vi "Test Copy from Pixmap Offset.vi"(8 "error in (no error)":errorcluster, 11 "Test Case In":refnum<class "Image.lvclass">) -> (0 "error out":errorcluster, 3 "Test Case Out":refnum<class "Image.lvclass">)   [LabVIEW 2020, in "g_ar_toolkit.test.lvlib" / "Image.lvclass"]
uses:
  Image.lvclass
  C:/Program Files (x86)/National Instruments/LabVIEW 2020/vi.lib/Astemes/LUnit/Test Case.lvclass
  g_ar_toolkit.image/ARGB Colour.ctl
  <vilib>/Astemes/LUnit/Test Case.lvclass/Test Case.ctl
  g_ar_toolkit.image/CreateEmptyImageARGB.vi
  g_ar_toolkit.image/CopyPixmapToImageFlattenMaskARGB.vi
  4993e8ee-a06a-463a-9684-69129f64d5ce.vi
  g_ar_toolkit.image/CreateEmptyImageARGB.vi/3321fa97-f432-4e1e-8db9-a0df79aed21b.vi
  g_ar_toolkit.image/CopyPixmapToImageFlattenMaskARGB.vi/80b1166a-8c06-443b-b271-eb6a715622f7.vi
  <vilib>/Astemes/LUnit/Append Pass Result.vi
  <vilib>/Astemes/LUnit/Append Fail Result.vi
  <vilib>/Astemes/LUnit/Describe Comparison.vi
  <vilib>/Astemes/LUnit/Compare Variants.vi
  g_ar_toolkit.image/FixPixmap.vi
  <vilib>/Astemes/LUnit/Run In UI.vi
  g_ar_toolkit.image/Default8bitColourMap.vi
  <vilib>/Utility/error.llb/Clear Errors.vi
  g_ar_toolkit.image/ARGBColourToU32.vi
  g_ar_toolkit.common/Module Path.vi
  <vilib>/Utility/error.llb/Error Cluster From Error Code.vi
  <vilib>/Astemes/LUnit/Describe Variant.vi
  g_ar_toolkit.image/g_ar_toolkit.image.lvlib
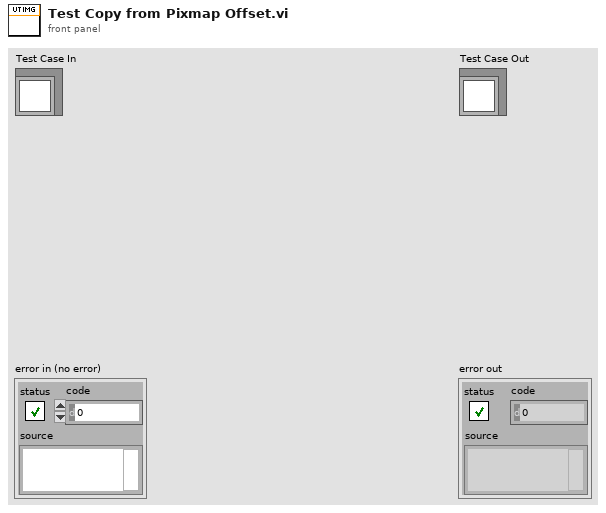
[diagram p1: front panel]
types:
  T1 = cluster{"Width":i16, "Style":enum32{"Solid", "Dash", "Dot", "DashDot", "DashDotDot"}}
  T2 = typedef "g_ar_toolkit.image.lvlib/ARGB Colour.ctl" = cluster{"Alpha":u8, "RGB":u32}
  T3 = cluster{"left":i16, "top":i16, "right":i16, "bottom":i16}
  T4 = typedef "imagedata.ctl" = cluster{"image type":i32, "image depth":i32, "image":u8[], "mask":u8[], "colors":u32[], "Rectangle":cluster{"left":i16, "top":i16, "right":i16, "bottom":i16}}
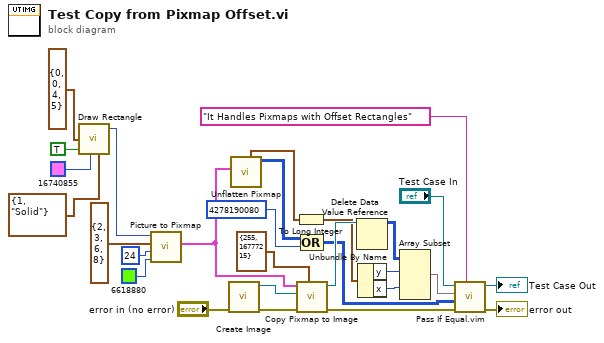
[diagram p0: block diagram]
diagram:
  n1 = call <vilib>:"Draw Rectangle.vi"("rect"=T3 {"left"=0, "top"=0, "right"=4, "bottom"=5}, "fill?(F)"=TRUE, "color(black)"=u32 16740855, "pen"=T1 {"Width"=1, "Style"=enum."Solid"}) -> ("new picture"=w24:picture)  [unwired: 5 in]
  n2 = call <vilib>:"Picture to Pixmap.vi"("Background Color"=u32 6618880, "depth"=24, "rect"=T3 {"left"=2, "top"=3, "right"=6, "bottom"=8}, "picture"=w24) -> ("image data"=w15:T4)  [unwired: 6 in, 1 out]
  n3 = call-poly "Create Image.vi"("error in (no error)"="error in (no error)") -> ("error out"=w3:errorcluster, "New ARGB Image"=w19:refnum<data-value>)  [unwired: 9 in]
  n4 = call <vilib>:"Unflatten Pixmap.vi"("image data"=w15) -> ("24-bit pixmap"=w8:u32[][], "top left"=w12:cluster{"x":i16, "y":i16})  [unwired: 4 in, 5 out]
  n5 = To Long Integer(number=w12) -> (32bit integer=w9:cluster{"x":i32, "y":i32})
  n6 = call-poly "Copy Pixmap to Image.vi"("Colour (Default: Black)"=T2 {"Alpha"=255, "RGB"=16777215}, "error in (no error)"=w3, "ARGB Image Destination"=w19, "Pixmap Image Data"=w15) -> ("error out"=w2:errorcluster, "ARGB Image Destination (duplicate)"=w14:refnum<data-value>)  [unwired: 6 in]
  n7 = Compound Arithmetic op=OR(w8, u32 4278190080) -> (w6:u32[][])
  n8 = Delete Data Value Reference(data value reference=w14) -> (data value=w13:u32[][])  [unwired: 1 in, 1 out]
  n9 = Unbundle By Name(w9) -> ("y"=w11:i32, "x"=w10:i32)
  n10 = Array Subset(array=w13, index (row)=w11, index (col)=w10) -> (w5:u32[][])  [unwired: 2 in]
  n11 = call "Pass If Equal.vim"("Description"="It Handles Pixmaps with Offset Rectangles", "error in (no error)"=w2, "Actual"=w6, "Expected"=w5, "LUnit Test Case In"="Test Case In") -> ("error out"=→"error out":errorcluster, "LUnit Test Case Out"=→"Test Case Out":refnum<class "Image.lvclass">)  [unwired: 5 in]
